vi "demo_.raverse.vi"() -> ()   [LabVIEW 2021]
panel:
  out "all data out":i32[](array[numeric])
  in  "Tree":string(tree)
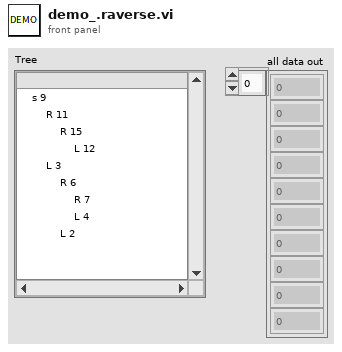
[diagram p1: front panel]
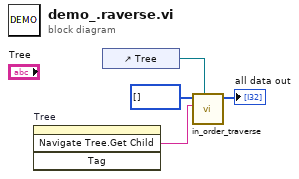
[diagram p0: block diagram]
diagram:
  n1 = invoke on="Tree" class="Tree (strict)" method="Navigate Tree.Get Child"() -> ("Navigate Tree:Get Child"=w3:string)  [unwired: 4 in, 3 out]
  n2 = control-ref of="Tree"() -> (w4:refnum<vi>)
  n3 = call "in_order_traverse.vi"("tree"=w4, "node"=w3, "all data"=i32[] []) -> ("all data out"=→"all data out":i32[])  [unwired: 7 in, 1 out]
